vi "Attenuator Initialize Graphs.vi"(8 "Attenuator Test Parameters":T1={"Stimulus"={"ATT Stimulus"={"Normalize"=TRUE, "Value (dB)"=0.0}, "VNA Stimulus"={"Use Instrument Settings"=FALSE, "Blank Frequencies"=FALSE, "Sweep Type"=enum."Linear", "Sweep"={"Fstart"=500.0, "Fstop"=1500.0, "Units"=enum."MHz", "Points"=201}, "Power (dBm)"=999.0, "IFBW (Hz)"=-1.0, "Sweep Time (s)"=-1.0, "Calibration"={"State"=FALSE, "String"=""}}}, "Measurement"={"Step (dB)"=enum."0.25", "Start (dB)"=0.0, "Stop (dB)"=31.75}, "Limit"={"Maximum Error"=0.3}, "Normalization"={"Normalized?"=FALSE, "Normalization Values (dB)"=[]}} {"Stimulus"."VNA Stimulus"."Sweep Time (s)" format="%.3g"}, 10 "Attenuation Variance":refnum<vi>, 11 "Frequency":refnum<vi>) -> ()   [LabVIEW 2011]
uses:
  TypeDefs/Attenuator Test Parameters.ctl
  TypeDefs/Attenuator Stimulus Parameters.ctl
  TypeDefs/Attenuator ATT Stimulus.ctl
  TypeDefs/Attenuator VNA Stimulus.ctl
  S Parameter/TypeDefs/SP Frequency Units.ctl
  TypeDefs/Attenuator VNA Calibration State.ctl
  TypeDefs/Attenuator Measurement Cluster.ctl
  TypeDefs/Attenuator Limit.ctl
  TypeDefs/Attenuator Calibration State.ctl
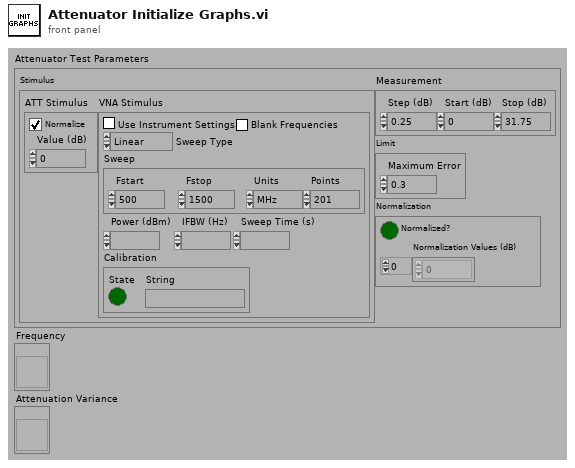
[diagram p1: front panel]
types:
  T1 = typedef "Attenuator Test Parameters.ctl" = cluster{"Stimulus":T2, "Measurement":T7, "Limit":T8, "Normalization":T9}
  T2 = typedef "Attenuator Stimulus Parameters.ctl" = cluster{"ATT Stimulus":T3, "VNA Stimulus":T4}
  T3 = typedef "Attenuator ATT Stimulus.ctl" = cluster{"Normalize":bool, "Value (dB)":dbl}
  T4 = typedef "Attenuator VNA Stimulus.ctl" = cluster{"Use Instrument Settings":bool, "Blank Frequencies":bool, "Sweep Type":enum32{"Linear", "Logarithmic", "List", "Power", "CW"}, "Sweep":cluster{"Fstart":dbl, "Fstop":dbl, "Units":T5, "Points":i32}, "Power (dBm)":dbl, "IFBW (Hz)":dbl, "Sweep Time (s)":dbl, "Calibration":T6}
  T5 = typedef "SP Frequency Units.ctl" = enum16{"Hz", "kHz", "MHz", "GHz", "Points"}
  T6 = typedef "Attenuator VNA Calibration State.ctl" = cluster{"State":bool, "String":string}
  T7 = typedef "Attenuator Measurement Cluster.ctl" = cluster{"Step (dB)":enum16{"0.25", "0.50", "1.00"}, "Start (dB)":dbl, "Stop (dB)":dbl}
  T8 = typedef "Attenuator Limit.ctl" = cluster{"Maximum Error":dbl}
  T9 = typedef "Attenuator Calibration State.ctl" = cluster{"Normalized?":bool, "Normalization Values (dB)":dbl[]}
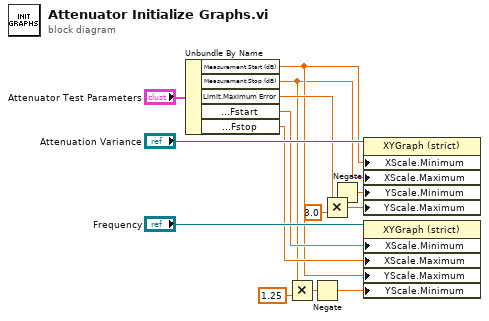
[diagram p0: block diagram]
diagram:
  n1 = Unbundle By Name("Attenuator Test Parameters") -> ("Measurement.Start (dB)"=w5:dbl, "Measurement.Stop (dB)"=w3:dbl, "Limit.Maximum Error"=w12:dbl, "Stimulus.VNA Stimulus.Sweep.Fstart"=w7:dbl, "Stimulus.VNA Stimulus.Sweep.Fstop"=w6:dbl)
  n2 = Multiply(x=w3, y=1.25) -> (x*y=w4:dbl)
  n3 = Negate(x=w4) -> (-x=w1:dbl)
  n4 = Multiply(x=w12, y=3.0) -> (x*y=w9:dbl)
  n5 = Negate(x=w9) -> (-x=w10:dbl)
  n6 = property class="XYGraph (strict)"(reference="Attenuation Variance", "XScale.Minimum"=w5, "XScale.Maximum"=w3, "YScale.Minimum"=w10, "YScale.Maximum"=w9) -> ()  [unwired: 1 in, 2 out]
  n7 = property class="XYGraph (strict)"(reference="Frequency", "XScale.Minimum"=w7, "XScale.Maximum"=w6, "YScale.Maximum"=w5, "YScale.Minimum"=w1) -> ()  [unwired: 1 in, 2 out]
